vi "Get Status.vi"(8 "error in (no error)":errorcluster, 11 "Interaction By Refererence in":refnum<class "Interaction By Refererence.lvclass">) -> (0 "error out":errorcluster, 2 "Status":string, 3 "Interaction By Refererence out":refnum<class "Interaction By Refererence.lvclass">)   [LabVIEW 2013, in "Interaction By Refererence.lvclass"]
uses:
  Interaction By Refererence.lvclass
  IObject.lvclass
  Interaction By Refererence.lvclass/Interaction By Refererence.ctl
  IContainer/Interaction/Interaction.lvclass
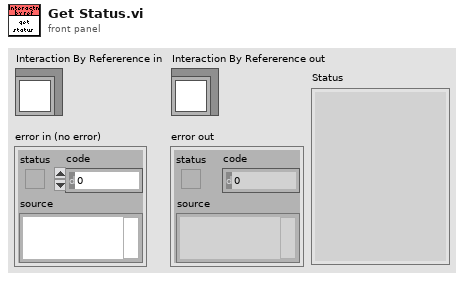
[diagram p1: front panel]
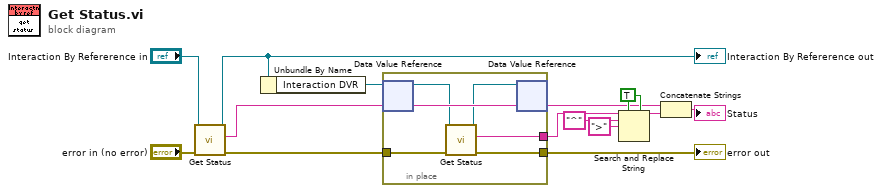
[diagram p0: block diagram]
diagram:
  w3 = TRUE ("replace all? (F)")
  n1 = call-parent "Get Status.vi"("error in (no error)"="error in (no error)", "IObject in"="Interaction By Refererence in") -> ("error out"=w10:errorcluster, "Status"=w1:string, "IObject out"=w8:refnum<class "Interaction By Refererence.lvclass">)  [unwired: 7 in]
  "Interaction By Refererence out" <- w8
  n2 = Unbundle By Name(w8) -> ("Interaction DVR"=w11:refnum<data-value>)
  n3 = in-place {
    in-place-border: [w18] -> w13
    in-place-border: [w17] -> w5
    in-place-border: w10 -> [w16]
    n4 = in-place-dvr #1(w11) -> (w15:refnum<class "Interaction.lvclass">)  [unwired: 1 out]
    n5 = call-dynamic "Get Status.vi"("error in (no error)"=w16, "IContainer in"=w15) -> ("error out"=w18:errorcluster, "Status"=w17:string, "IContainer out"=w14:refnum<class "Interaction.lvclass">)  [unwired: 7 in]
    n6 = in-place-dvr #1(w14) -> ()  [unwired: 2 out]
  }
  "error out" <- w13
  n7 = Search and Replace String(replace all?=w3, multiline?=w3, input string=w5, search string="^", replace string=">" ("replace string (\"\")")) -> (result string=w4:string)  [unwired: 3 in, 3 out]
  n8 = Concatenate Strings(w1, w4) -> (→"Status":string)
